vi "Run Robot Routine.vi"(8 "error in (no error)":errorcluster, 11 "Robot in":refnum<class "Robot.lvclass">) -> (0 "error out":errorcluster, 3 "Robot out":refnum<class "Robot.lvclass">)   [LabVIEW 2018, in "Robot.lvlib" / "Robot.lvclass"]
uses:
  Robot.lvclass
  Robot.lvclass/Robot.ctl
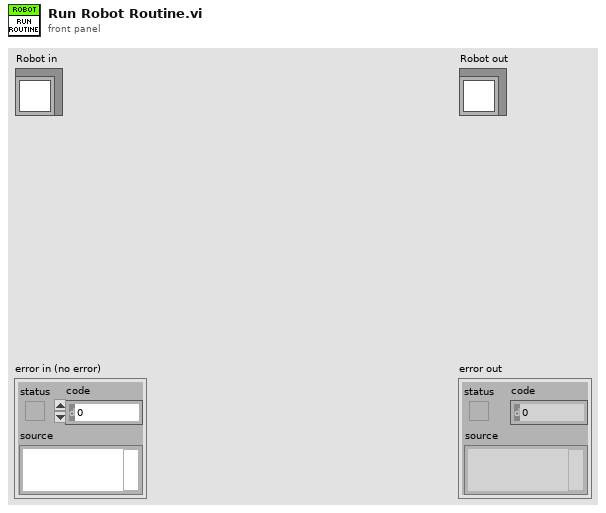
[diagram p1: front panel]
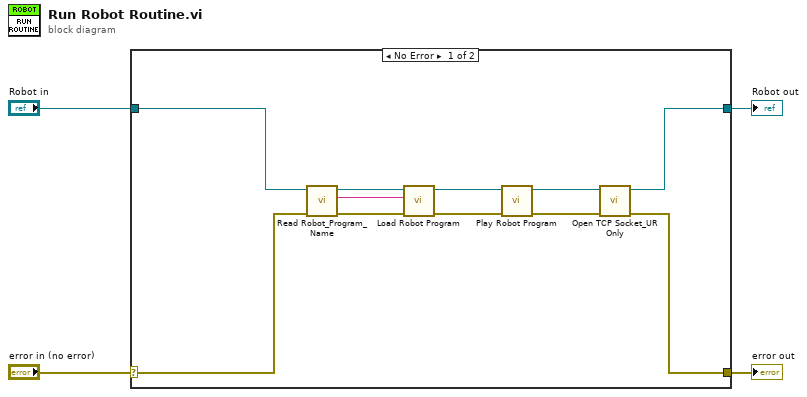
[diagram p0: block diagram]
diagram:
  n1 = case shown="No Error" "error in (no error)" {
    selector: "error in (no error)" -> [w13 w17]
    tunnel: [w7 w17] -> w3
    tunnel: [w5 w16] -> w1
    tunnel: "Robot in" -> [w11 w16]
    frame No Error {
      n2 = call "Read Robot_Program_Name.vi"("error in (no error)"=w13, "Robot in"=w11) -> ("error out"=w12:errorcluster, "Robot_Program_Name"=w9:string, "Robot out"=w10:refnum<class "Robot.lvclass">)  [unwired: 7 in]
      n3 = call-dynamic "Load Robot Program.vi"("error in (no error)"=w12, "Program_Name"=w9, "Robot in"=w10) -> ("error out"=w14:errorcluster, "Robot out"=w15:refnum<class "Robot.lvclass">)  [unwired: 7 in]
      n4 = call-dynamic "Play Robot Program.vi"("error in (no error)"=w14, "Robot in"=w15) -> ("error out"=w8:errorcluster, "Robot out"=w6:refnum<class "Robot.lvclass">)  [unwired: 8 in]
      n5 = call-dynamic "Open TCP Socket_UR Only.vi"("error in (no error)"=w8, "Robot in"=w6) -> ("error out"=w7:errorcluster, "Robot out"=w5:refnum<class "Robot.lvclass">)  [unwired: 8 in]
    }
    frame Error {
    }
  }
  "error out" <- w3
  "Robot out" <- w1
